vi "Signal(Float64)ToNode(viaString).vi"(0 "Tree DVR in":refnum<data-value>, 1 "NodePath":string, 2 "y-axis (Data Range)":dbl[](array[numeric]), 3 "Start Time":dbl, 4 "Delta t":dbl, 5 "Error in":errorcluster) -> (6 "Tree DVR out":refnum<data-value>, 8 "Error out":errorcluster)   [LabVIEW 2014]
uses:
  <vilib>/MDSplus/Classes/Tree_Class/Tree.lvclass
  <vilib>/MDSplus/Library/MDSplus.lvlib
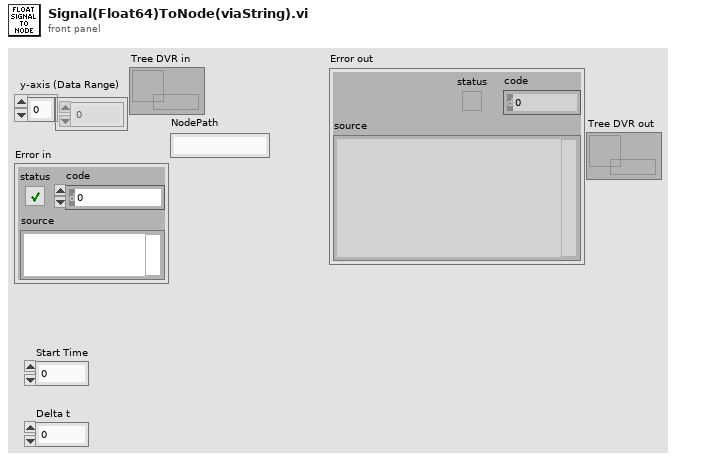
[diagram p1: front panel]
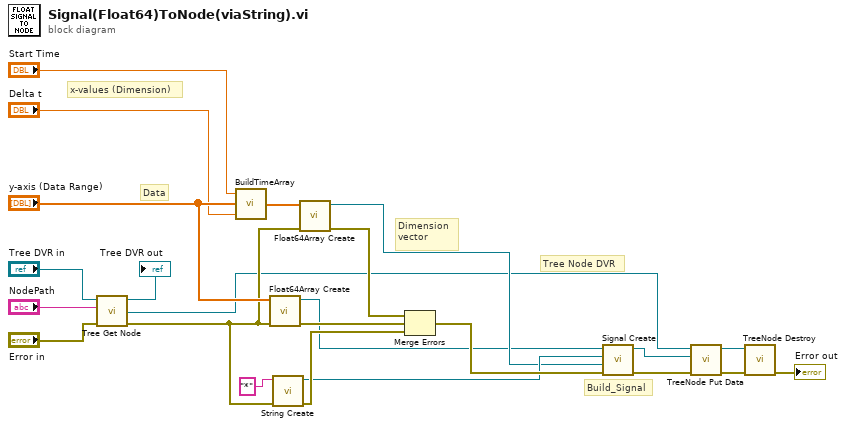
[diagram p0: block diagram]
diagram:
  # "Build_Signal"
  # "Dimension vector"
  # "x-values (Dimension)"
  # "Tree Node DVR"
  # "Data"
  n1 = call <vilib>:"Tree Get Node.vi"("error in (no error)"="Error in", "Path"="NodePath", "Tree DVR in"="Tree DVR in") -> ("error out"=w9:errorcluster, "Node out"=w4:refnum<data-value>, "Tree DVR out"=→"Tree DVR out":refnum<data-value>)  [unwired: 6 in]
  n2 = call "BuildTimeArray.vi"("Time Increment (dt)"="Delta t", "Data Array (y-values)"="y-axis (Data Range)", "Start Time (t_o)"="Start Time") -> ("Time Array (x-values)"=w13:dbl[])
  n3 = call <vilib>:"Float64Array Create.vi"("error in (no error)"=w9, "DBL array in"="y-axis (Data Range)") -> ("error out"=w18:errorcluster, "Float64Array DVR out"=w6:refnum<data-value>)  [unwired: 8 in]
  n4 = call <vilib>:"String Create.vi"("error in (no error)"=w9, "String value in"="*") -> ("error out"=w10:errorcluster, "String DVR out"=w8:refnum<data-value>)  [unwired: 8 in]
  n5 = call <vilib>:"Float64Array Create.vi"("error in (no error)"=w9, "DBL array in"=w13) -> ("error out"=w12:errorcluster, "Float64Array DVR out"=w7:refnum<data-value>)  [unwired: 8 in]
  n6 = Merge Errors(w12, w18, w10) -> (w17:errorcluster)
  n7 = call <vilib>:"Signal Create.vi"("error in (no error)"=w17, "Dimension"=w7, "Raw"=w8, "Data"=w6) -> ("error out"=w19:errorcluster, "Signal DVR out"=w5:refnum<data-value>)  [unwired: 6 in]
  n8 = call <vilib>:"TreeNode Put Data.vi"("error in (no error)"=w19, "Data"=w5, "TreeNode DVR in"=w4) -> ("error out"=w1:errorcluster, "TreeNode DVR out"=w2:refnum<data-value>)  [unwired: 7 in]
  n9 = call <vilib>:"TreeNode Destroy.vi"("error in (no error)"=w1, "TreeNode DVR in"=w2) -> ("error out"=→"Error out":errorcluster)  [unwired: 9 in]
